vi "Get Alias Mappings.vi"(8 "error in (no error)":errorcluster, 11 "Aliases Ref in":T2 format="%.0x") -> (0 "error out":errorcluster, 2 "Alias Mappings":T1[](array[typedef]), 3 "Aliases Ref out":T2 format="%.0x")   [LabVIEW 2017, in "Switch Scripting.lvlib"]
uses:
  Switch Scripting.lvlib
  <vilib>/NI Veristand/Custom Device API/Custom Device Item Ref.ctl
  Shared/Alias Mapping.ctl
  <vilib>/NI VeriStand/Custom Device API/Custom Device API.lvlib
  Shared/Routing and Faulting Shared.lvlib
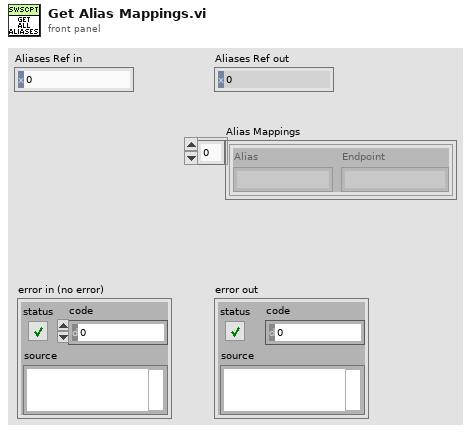
[diagram p1: front panel]
types:
  T1 = typedef "Routing and Faulting Shared.lvlib/Alias Mapping.ctl" = cluster{"Alias":string, "Endpoint":string}
  T2 = typedef "Custom Device API.lvlib/Custom Device Item Ref.ctl" = u64
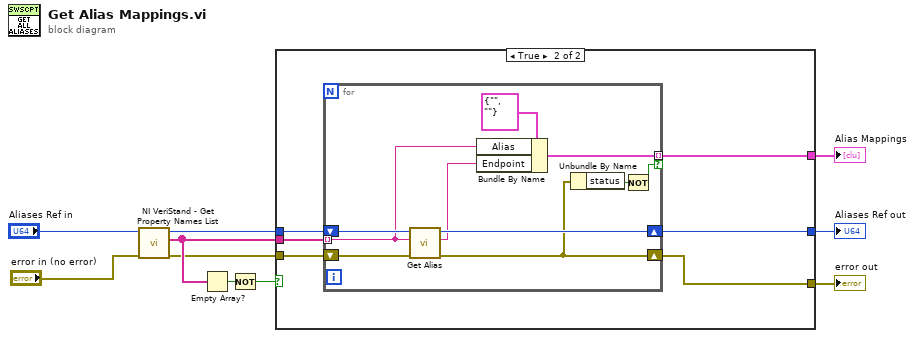
[diagram p0: block diagram]
diagram:
  n1 = call <vilib>:"NI VeriStand - Get Property Names List.vi"("error in (no error)"="error in (no error)", "Item Ref in"="Aliases Ref in") -> ("error out"=w8:errorcluster, "Property Names"=w9:string[], "Item Ref out"=w4:T2)  [unwired: 7 in]
  n2 = Empty Array?(array=w9) -> (empty?=w10:bool)
  n3 = Not(x=w10) -> (.not. x?=w2:bool)
  n4 = case shown="True" w2 {
    tunnel: w9 -> [_ w18]
    tunnel: w8 -> [w11 w17]
    tunnel: [w11 w16] -> w6
    tunnel: w4 -> [w12 w15]
    tunnel: [w12 w14] -> w3
    tunnel: [_ w13] -> w1
    frame False {
    }
    frame True {
      n5 = for {
        tunnel: w18 -> [w24] mode=indexing
        shift-right: [w21] -> w16
        shift-left: w17 -> [w26]
        tunnel: [w22] -> w13 mode=indexing if=w19
        shift-right: [w27] -> w14
        shift-left: w15 -> [w28]
        n6 = call "Get Alias.vi"("error in (no error)"=w26, "Alias"=w24, "Aliases Ref in"=w28) -> ("error out"=w21:errorcluster, "Endpont"=w23:string, "Aliases Ref out"=w27:T2)  [unwired: 6 in]
        n7 = Bundle By Name(cluster=T1 {"Alias"="", "Endpoint"=""} ("Alias Mapping"), "Alias"=w24, "Endpoint"=w23) -> (w22:T1)
        n8 = Unbundle By Name(w21) -> ("status"=w20:bool)
        n9 = Not(x=w20) -> (.not. x?=w19:bool)
      }
    }
  }
  "error out" <- w6
  "Aliases Ref out" <- w3
  "Alias Mappings" <- w1
